vi "InlineReferencePool.vi"(6 "functions":T1, 8 "error in (no error)":errorcluster, 9 "inline vi ref":refnum<vi>) -> (0 "error out":errorcluster, 2 "All actor refs":refnum<vi>[](array[refnum]))   [LabVIEW 2021, in "YActor.lvclass"]
uses:
  YActor.lvclass
  InlineReferencePool.ctl
  private/ActorPoolFunctions.ctl
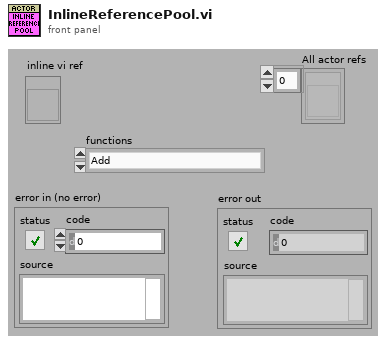
[diagram p1: front panel]
types:
  T1 = typedef "YActor.lvclass/InlineReferencePool.ctl" = enum16{"Add", "ClearAll?"}
  T2 = typedef "YActor.lvclass/ActorPoolFunctions.ctl" = enum16{"Add", "GetAll", "Delete"}
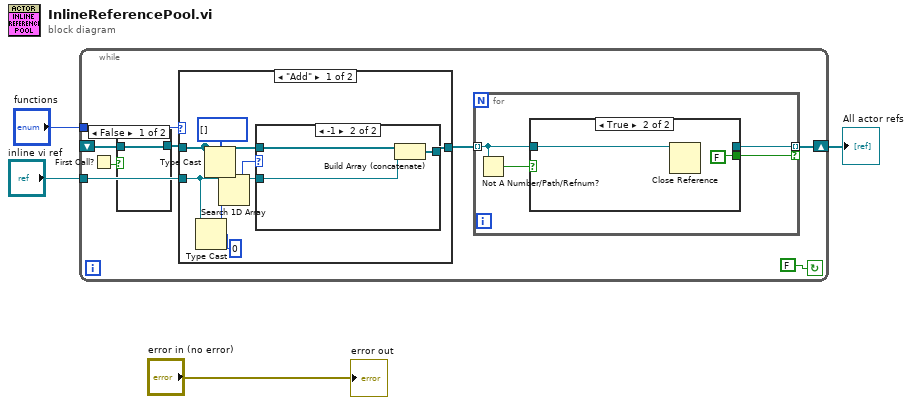
[diagram p0: block diagram]
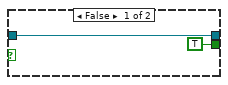
[diagram p3: hidden frame]
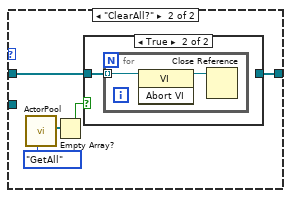
[diagram p5: hidden frame]
diagram:
  n1 = while {
    tunnel: "functions" -> [w12]
    shift-right: [w9] -> w2
    shift-left: _ -> [w6]
    tunnel: "inline vi ref" -> [w10]
    stop <- FALSE continue-if-true
    n2 = First Call?() -> (First Call?: T/F=w7:bool)
    n3 = case shown="False" w7 {
      tunnel: [w13 _] -> w5
      tunnel: w6 -> [w13 _]
      frame False {
      }
      frame True {
      }
    }
    n4 = case shown="\"Add\"" w12 {
      tunnel: w5 -> [w28 w35]
      tunnel: [w29 w34] -> w8
      tunnel: w10 -> [w27 _]
      frame "Add" {
        n5 = Type Cast(type=0, x=w27) -> (*(type *) &x=w23:i32)
        n6 = Type Cast(type=i32[] [], x=w28) -> (*(type *) &x=w24:i32[])
        n7 = Search 1D Array(1D array=w24, element=w23) -> (index of element=w22:i32)  [unwired: 1 in]
        n8 = case shown="-1" w22 {
          tunnel: [w30 w33] -> w29
          tunnel: w28 -> [w30 w32]
          tunnel: w27 -> [_ w31]
          frame 0, Default {
          }
          frame -1 {
            n9 = Build Array (concatenate)(w32, w31) -> (w33:refnum<vi>[])
          }
        }
      }
      frame "ClearAll?" {
        n10 = call "ActorPool.vi"("Functions"=ActorPoolFunctions."GetAll" ("functions")) -> ("AllActorRefs"=w37:refnum<vi>[])  [unwired: 8 in, 2 out]
        n11 = Empty Array?(array=w37) -> (empty?=w36:bool)
        n12 = case shown="True" w36 {
          tunnel: [w39 _] -> w34
          tunnel: w35 -> [w39 w40]
          frame False {
          }
          frame True {
            n13 = for {
              tunnel: w40 -> [w42] mode=indexing
              n14 = invoke class="VI" method="Abort VI"(reference=w42) -> (reference out=w41:refnum<vi>)  [unwired: 2 in, 2 out]
              n15 = Close Reference(reference=w41) -> ()  [unwired: 1 in, 1 out]
            }
          }
        }
      }
    }
    n16 = for {
      tunnel: w8 -> [w15] mode=indexing
      tunnel: [w14] -> w9 mode=indexing if=w16
      n17 = Not A Number/Path/Refnum?(number/path/refnum=w15) -> (NaN/Path/Refnum?=w17:bool)
      n18 = case shown="True" w17 {
        tunnel: w15 -> [w19 w21]
        tunnel: [TRUE FALSE] -> w16
        tunnel: [w19 _] -> w14
        frame False {
        }
        frame True {
          n19 = Close Reference(reference=w21) -> ()  [unwired: 1 in, 1 out]
        }
      }
    }
  }
  "All actor refs" <- w2
  "error out" <- "error in (no error)"
